vi "Simple Edge Detection (Rising).vi"(11 "Current Bit":bool=TRUE) -> (3 "Rising Edge found?":bool)   [LabVIEW 2022 SP3, in "hse-misc.lvlib"]
doc: "Returns True if a rising edge (False -> True) occures.\n\n(This VI is inlined.)\n\n____\nHAMPEL SOFTWARE ENGINEERING v3.8.0 (2023-12-18 14:41)"
uses:
  hse-misc.lvlib
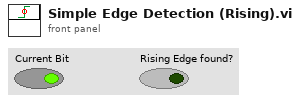
[diagram p1: front panel]
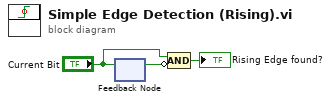
[diagram p0: block diagram]
diagram:
  n1 = feedback #1() -> (w3:bool)  [unwired: 1 in]
  n2 = feedback-in #1("Current Bit") -> ()
  n3 = Compound Arithmetic op=AND("Current Bit", invert w3) -> (→"Rising Edge found?":bool)
